vi "close.vi"(8 "error in (no error)":errorcluster, 11 "CNT90 in":refnum<class "CNT90.lvclass">) -> (0 "error out":errorcluster, 3 "CNT90 out":refnum<class "CNT90.lvclass">)   [LabVIEW 2019, in "CNT90.lvclass"]
uses:
  CNT90.lvclass
  CNT90.lvclass/CNT90.ctl
  <instrlib>/Pendulum CNT90/Pendulum CNT90.lvlib
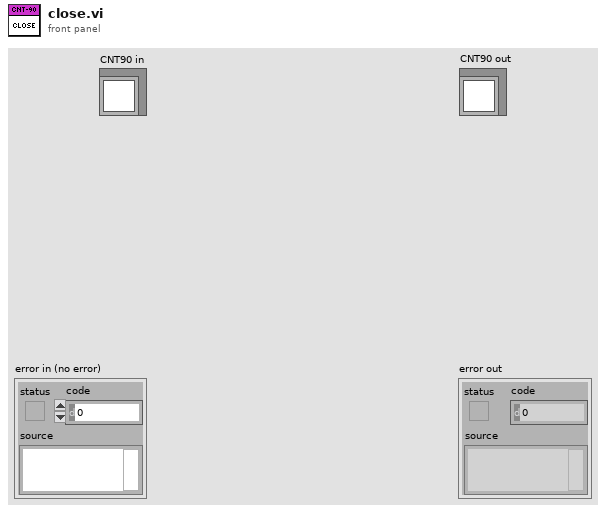
[diagram p1: front panel]
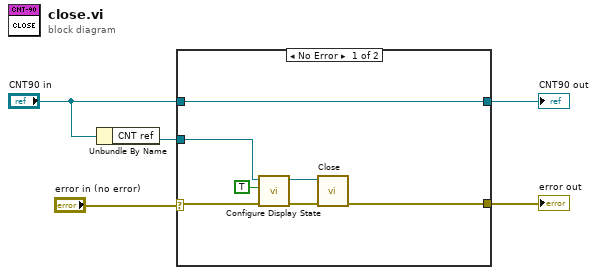
[diagram p0: block diagram]
diagram:
  n1 = Unbundle By Name("CNT90 in") -> ("CNT ref"=w1:refnum<visa-resource-name>)
  n2 = case shown="No Error" "error in (no error)" {
    selector: "error in (no error)" -> [w8 w14]
    tunnel: [w7 w14] -> w4
    tunnel: [w12 w13] -> w3
    tunnel: "CNT90 in" -> [w12 w13]
    tunnel: w1 -> [w6 _]
    frame No Error {
      n3 = call <instrlib>:"Configure Display State.vi"("error in (no error)"=w8, "Display State (T: On)"=TRUE, "VISA resource name"=w6) -> ("error out"=w11:errorcluster, "VISA resource name out"=w10:refnum<visa-resource-name>)  [unwired: 7 in]
      n4 = call <instrlib>:"Close.vi"("error in (no error)"=w11, "VISA resource name"=w10) -> ("error out"=w7:errorcluster)  [unwired: 9 in]
    }
    frame Error {
    }
  }
  "error out" <- w4
  "CNT90 out" <- w3
